vi "daq calib.vi"() -> ()   [LabVIEW 2010]
doc: "I. Description:\nThis example demonstrates how to take a single Measurement (Sample) from an Analog Input Channel.\n\nII. Instructions for Running:\n1. Select the Physical Channel to correspond to where your signal is input on the DAQ device.\n2. Enter the Minimum and Maximum Voltage Ranges\nNote: For better accuracy try to match the Input Ranges to the expected voltage level of the measured signal.\nNote: Use the Gen Voltage Update example to provide a signal on your DAQ device to measure.\n\nIII. Block Diagram Steps:\n1. Create an Analog Input Voltage Channel.\n2. Use the Read VI to Measure 1 Sample from 1 Channel on the Data\nAcquisition Card. Set a timeout so an error is returned if the sample\nis not returned in the specified time limit\n3. Call the Clear Task VI to clear the Task.\n4. Use the popup dialog box to display an error if any.\n\nIV. I/O Connections Overview:\nMake sure your signal input terminal matches the Physical Channel I/O Control."
uses:
  <vilib>/sound2/lvsound2.llb/Sound Data Format.ctl
  <vilib>/Utility/error.llb/DialogType.ctl
  <vilib>/sound2/lvsound2.llb/Sound Output Task ID.ctl
  <vilib>/DAQmx/read.llb/DAQmx Read (Analog DBL 1Chan 1Samp).vi
  <vilib>/DAQmx/write.llb/DAQmx Write (Analog DBL 1Chan 1Samp).vi
  <vilib>/DAQmx/create/channels.llb/DAQmx Create Channel (AI-Voltage-Basic).vi
  <vilib>/DAQmx/create/channels.llb/DAQmx Create Channel (AO-Voltage-Basic).vi
  <vilib>/Utility/file.llb/Write To Spreadsheet File (DBL).vi
  <vilib>/daqmx/miscellaneous.llb/DAQmx Fill In Error Info.vi
  <vilib>/Analysis/NI_AALBase.lvlib
panel:
  out "Vez #":i32
  out "Paso #":i32
  in  "DAC Paso":dbl step=0.001 format="%0.3f"
  in  "DAC Hasta":dbl step=0.001 format="%0.3f"
  in  "DAC Desde":dbl step=0.001 format="%0.3f"
  in  "tiempo entre pasos (ms)":dbl
  in  "Sound Paso":dbl step=0.001 format="%0.3f"
  in  "Sound Hasta":dbl step=0.001 format="%0.3f"
  in  "Sound Desde":dbl step=0.001 format="%0.3f"
  in  "DAC (T) / Sound (F)":bool
  in  "Sound Controls":T2={"device ID"=0, "sound format"={"sample rate (S/s)"=44000.0, "number of channels"=2, "bits per sample"=16}, "time (ms)"=200.0}
  out "Numeric":u32
  in  "Corre":bool
  in  "N":i32
  in  "Maximum Value 2":dbl=10.0 caption="Maximum Value" format="%.2f"
  in  "Minimum Value 2":dbl=-10.0 caption="Minimum Value" format="%0.2f"
  out "In Range?":bool
  in  "Physical Channel 2":tag="Dev1/ai0" caption="Physical Channel"
  in  "stop":bool
  in  "Maximum Value":dbl=10.0 format="%.2f"
  in  "Minimum Value":dbl=-10.0 format="%0.2f"
  in  "Physical Channel":tag="Dev1/ai0"
  # "Channel Parameters"
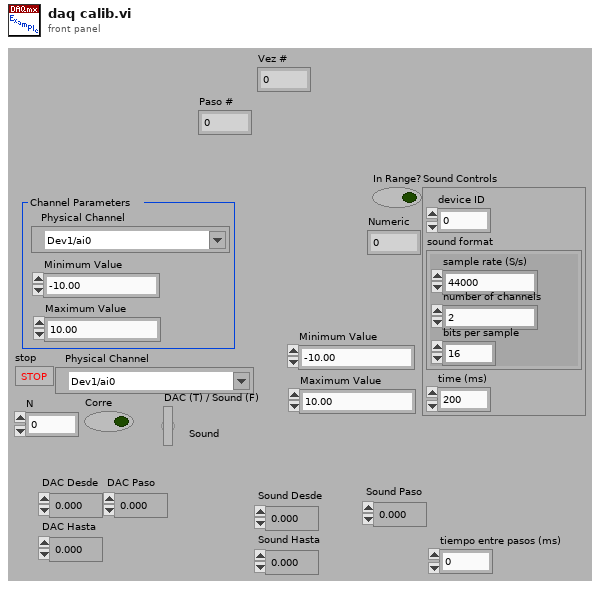
[diagram p1: front panel]
types:
  T1 = typedef "Sound Data Format.ctl" = cluster{"sample rate (S/s)":dbl, "number of channels":i32, "bits per sample":i32}
  T2 = cluster{"device ID":u32, "sound format":T1, "time (ms)":dbl}
  T3 = typedef "Sound Output Task ID.ctl" = u32
  T4 = cluster{"task ID":T3, "error":errorcluster, "sound format":T1}
  T5 = typedef "DialogType.ctl" = u16
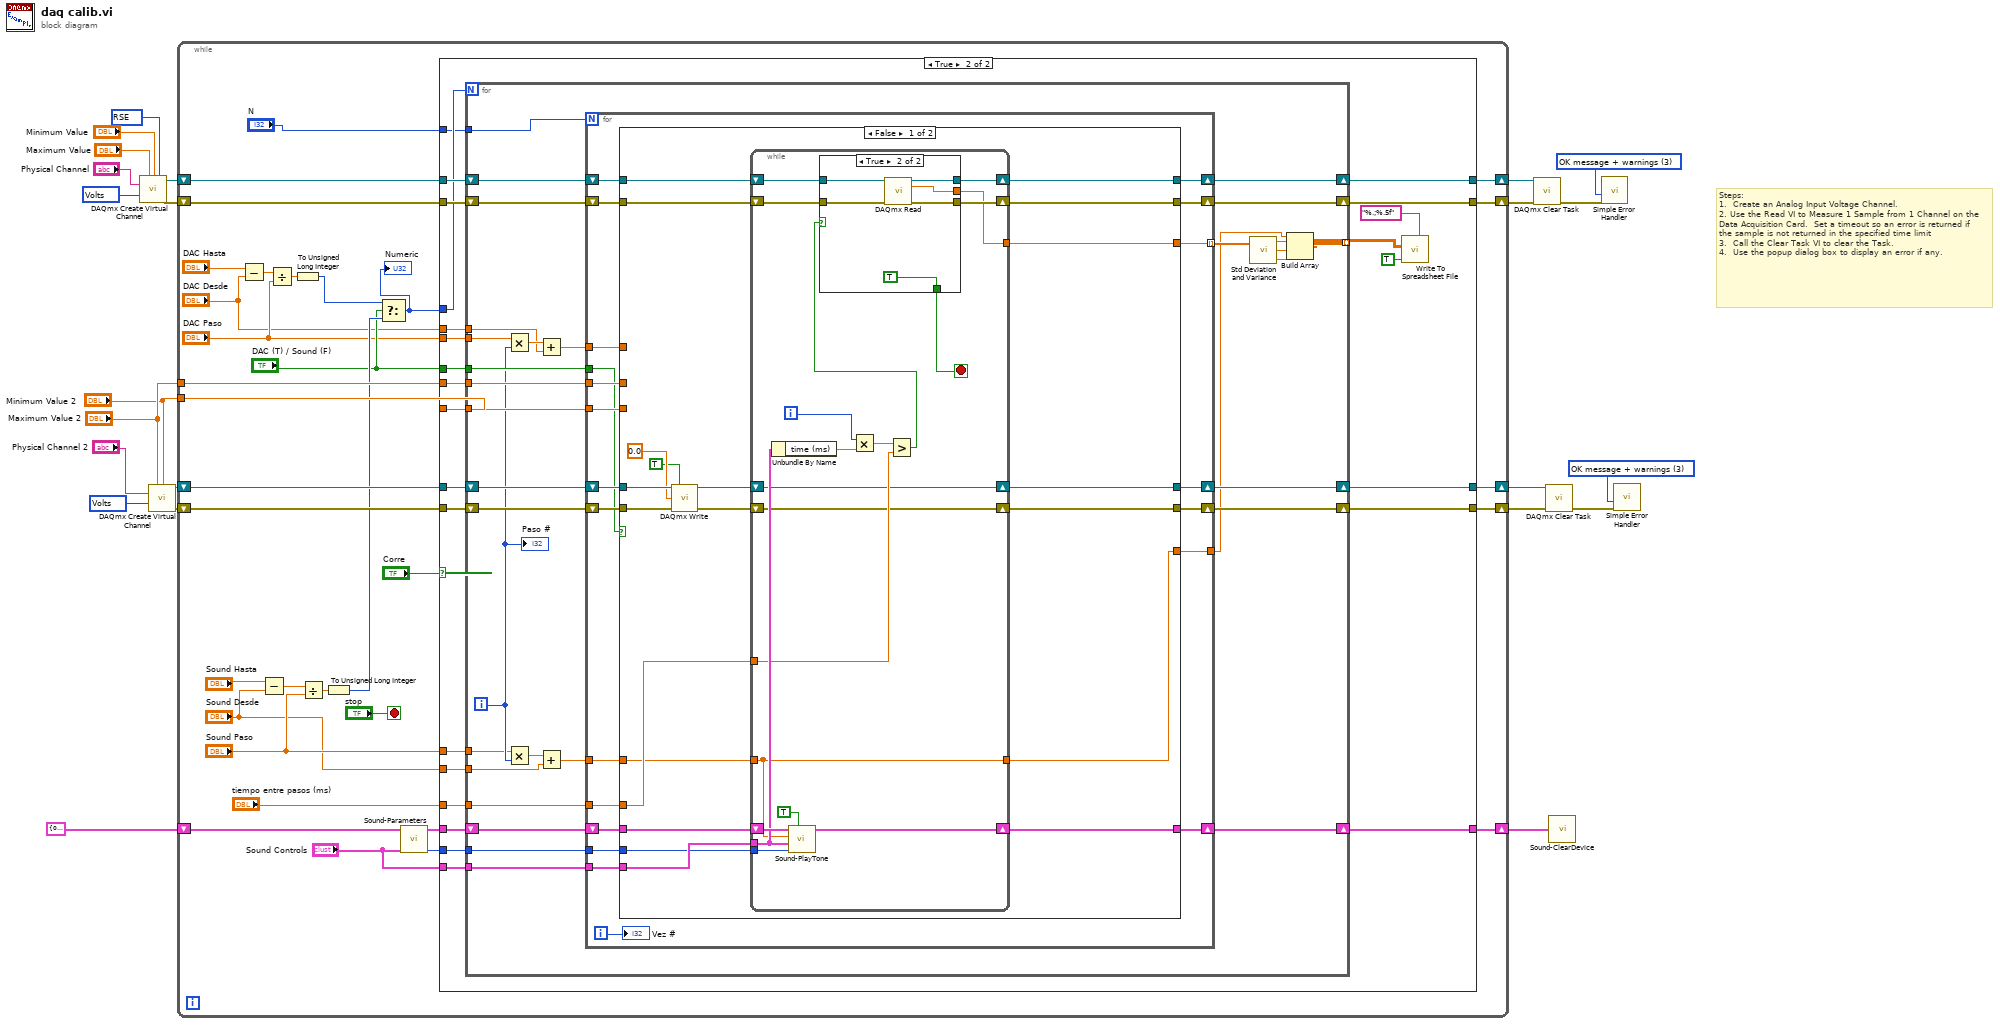
[diagram p0: block diagram]
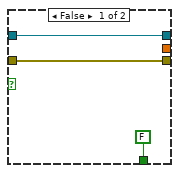
[diagram p3: hidden frame]
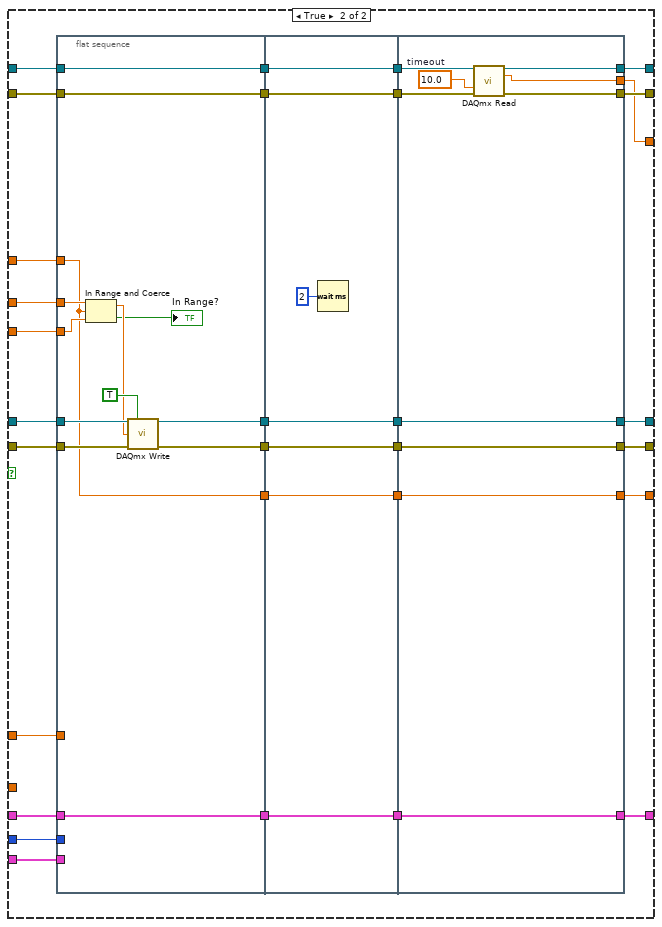
[diagram p4: hidden frame]
diagram:
  w5 = 10083 items=["default"=-1, "RSE"=10083, "NRSE"=10078, "Differential"=10106, "Pseudodifferential"=12529] ("input terminal configuration")
  w8 = 10348 items=["Volts"=10348, "From Custom Scale"=10065] ("units")
  w9 = 10348 items=["Volts"=10348, "From Custom Scale"=10065] ("units")
  w13 = T5 3 items=["no dialog", "OK message", "continue or stop message", "OK message + warnings", "continue/stop + warnings"] ("type of dialog (OK msg:1)")
  w20 = T5 3 items=["no dialog", "OK message", "continue or stop message", "OK message + warnings", "continue/stop + warnings"] ("type of dialog (OK msg:1)")
  # "Steps: \n1.  Create an Analog Input Voltage Channel. \n2. Use the Read VI to Measure 1 Sample from 1 Channel on the Data Acquisition Card.  Set a timeout so an error is returned if the sample is not returned in the specified time limit\n3.  Call the Clear Task VI to clear the Task.\n4.  Use the popup dialog box to display an error if any."
  n1 = call-poly <vilib>:"DAQmx Create Virtual Channel.vi"("maximum value"="Maximum Value", "minimum value"="Minimum Value", "input terminal configuration"=w5, "physical channels"="Physical Channel", "units"=w9) -> ("task out"=w22:refnum<k21>, "error out"=w21:errorcluster)  [unwired: 9 in]
  n2 = call-poly <vilib>:"DAQmx Create Virtual Channel.vi"("maximum value"="Maximum Value 2", "minimum value"="Minimum Value 2", "physical channels"="Physical Channel 2", "units"=w8) -> ("task out"=w15:refnum<k21>, "error out"=w14:errorcluster)  [unwired: 10 in]
  n3 = while {
    shift-right: [w50] -> w19
    shift-left: w22 -> [w53]
    shift-right: [w51] -> w18
    shift-left: w21 -> [w52]
    shift-right: [w49] -> w11
    shift-left: w15 -> [w55]
    shift-right: [w48] -> w10
    shift-left: w14 -> [w54]
    tunnel: "Maximum Value 2" -> [w47]
    tunnel: "Minimum Value 2" -> [w46]
    shift-right: [w42] -> w1
    shift-left: T4 {"task ID"=0, "error"={"status"=TRUE, "code"=0, "source"=""}, "sound format"={"sample rate (S/s)"=0.0, "number of channels"=0, "bits per sample"=0}} ("Sound Device OUT") -> [w44]
    stop <- "stop" stop-if-true
    n4 = Subtract(x="DAC Hasta", y="DAC Desde") -> (x-y=w29:dbl)
    n5 = Subtract(x="Sound Hasta", y="Sound Desde") -> (x-y=w38:dbl)
    n6 = Divide(x=w29, y="DAC Paso") -> (x/y=w28:dbl)
    n7 = To Unsigned Long Integer(number=w28) -> (unsigned 32bit integer=w27:u32)
    n8 = Divide(x=w38, y="Sound Paso") -> (x/y=w37:dbl)
    n9 = To Unsigned Long Integer(number=w37) -> (unsigned 32bit integer=w32:u32)
    n10 = Select(t=w27, s="DAC (T) / Sound (F)", f=w32) -> (s? t:f=w39:u32)
    "Numeric" <- w39
    n11 = call "Sound-Parameters.vi"("Sound Controls"="Sound Controls", "Sound Device IN"=w44) -> ("#samples"=w41:u32, "Sound Device OUT"=w43:T4)  [unwired: 3 in, 1 out]
    n12 = case shown="True" "Corre" {
      tunnel: w55 -> [w59 w86]
      tunnel: w54 -> [w58 w85]
      tunnel: w53 -> [w61 w84]
      tunnel: w52 -> [w60 w83]
      tunnel: [w60 w82] -> w51
      tunnel: [w61 w81] -> w50
      tunnel: [w59 w80] -> w49
      tunnel: [w58 w79] -> w48
      tunnel: w47 -> [_ w78]
      tunnel: w46 -> [_ w77]
      tunnel: w39 -> [_ w76]
      tunnel: "DAC Paso" -> [_ w75]
      tunnel: "DAC Desde" -> [_ w74]
      tunnel: "N" -> [_ w73]
      tunnel: "DAC (T) / Sound (F)" -> [_ w69]
      tunnel: w43 -> [w57 w68]
      tunnel: [w57 w67] -> w42
      tunnel: w41 -> [_ w66]
      tunnel: "Sound Controls" -> [_ w65]
      tunnel: "Sound Paso" -> [_ w64]
      tunnel: "Sound Desde" -> [_ w63]
      tunnel: "tiempo entre pasos (ms)" -> [_ w62]
      frame False {
      }
      frame True {
        n13 = for {
          N: w76 -> [_]
          tunnel: w78 -> [w110]
          tunnel: w77 -> [w109]
          shift-right: [w114] -> w82
          shift-left: w83 -> [w115]
          shift-right: [w113] -> w81
          shift-left: w84 -> [w116]
          shift-right: [w112] -> w80
          shift-left: w86 -> [w118]
          shift-right: [w111] -> w79
          shift-left: w85 -> [w117]
          tunnel: w75 -> [w107]
          tunnel: w74 -> [w106]
          tunnel: w73 -> [w105]
          tunnel: [w103] -> w72 mode=indexing
          tunnel: w69 -> [w97]
          shift-right: [w95] -> w67
          shift-left: w68 -> [w96]
          tunnel: w66 -> [w94]
          tunnel: w65 -> [w93]
          tunnel: w64 -> [w90]
          tunnel: w63 -> [w89]
          tunnel: w62 -> [w87]
          i -> [w91]
          n14 = Multiply(x=w107, y=w91) -> (x*y=w108:dbl)
          n15 = Multiply(x=w90, y=w91) -> (x*y=w92:dbl)
          n16 = Add(x=w108, y=w106) -> (x+y=w99:dbl)
          n17 = Add(x=w92, y=w89) -> (x+y=w88:dbl)
          n18 = for {
            N: w105 -> [_]
            tunnel: w110 -> [w131]
            tunnel: w109 -> [w130]
            shift-right: [w134] -> w113
            shift-left: w116 -> [w137]
            shift-right: [w135] -> w114
            shift-left: w115 -> [w136]
            shift-right: [w133] -> w112
            shift-left: w118 -> [w139]
            shift-right: [w132] -> w111
            shift-left: w117 -> [w138]
            tunnel: w99 -> [w129]
            tunnel: [w128] -> w102 mode=indexing
            tunnel: [w127] -> w98
            tunnel: w97 -> [w120]
            shift-right: [w125] -> w95
            shift-left: w96 -> [w126]
            tunnel: w94 -> [w124]
            tunnel: w93 -> [w123]
            tunnel: w88 -> [w122]
            tunnel: w87 -> [w121]
            i -> [w119]
            n19 = case shown="False" w120 {
              tunnel: w139 -> [w142 w205]
              tunnel: w138 -> [w143 w204]
              tunnel: w137 -> [w157 w203]
              tunnel: w136 -> [w155 w202]
              tunnel: [w154 w201] -> w135
              tunnel: [w156 w200] -> w134
              tunnel: [w147 w199] -> w133
              tunnel: [w148 w198] -> w132
              tunnel: w131 -> [_ w197]
              tunnel: w130 -> [_ w196]
              tunnel: w129 -> [_ w195]
              tunnel: [w149 w194] -> w128
              tunnel: [w146 w193] -> w127
              tunnel: w126 -> [w159 w192]
              tunnel: [w158 w191] -> w125
              tunnel: w124 -> [w152 w190]
              tunnel: w123 -> [w153 w189]
              tunnel: w122 -> [w150 w188]
              tunnel: w121 -> [w151 _]
              frame False {
                n20 = call-poly <vilib>:"DAQmx Write.vi"("task/channels in"=w142, "auto start"=TRUE, "data"=0.0, "error in"=w143) -> ("task out"=w145:refnum<k21>, "error out"=w144:errorcluster)  [unwired: 9 in, 1 out]
                n21 = while {
                  tunnel: w151 -> [w170]
                  tunnel: w150 -> [w160]
                  tunnel: w153 -> [w172]
                  tunnel: w152 -> [w174]
                  shift-right: [w175] -> w156
                  shift-left: w157 -> [w176]
                  shift-right: [w177] -> w158
                  shift-left: w159 -> [w178]
                  shift-right: [w167] -> w154
                  shift-left: w155 -> [w166]
                  tunnel: [w165] -> w149
                  shift-right: [w163] -> w147
                  shift-left: w145 -> [w163]
                  shift-right: [w164] -> w148
                  shift-left: w144 -> [w164]
                  tunnel: [w160] -> w146
                  i -> [w161]
                  stop <- w169 stop-if-true
                  n22 = Unbundle By Name(w172) -> ("time (ms)"=w162:dbl)
                  n23 = call "Sound-PlayTone.vi"("sound?"=TRUE ("DAQ?"), "# samples"=w174, "Sound Controls"=w172, "Frecuencia"=w160, "Sound Device IN"=w178) -> ("Sound Device OUT"=w177:T4)  [unwired: 3 in, 1 out]
                  n24 = Multiply(x=w161, y=w162) -> (x*y=w171:dbl)
                  n25 = Greater?(x=w171, y=w170) -> (0:w168:bool)
                  n26 = case shown="True" w168 {
                    tunnel: w176 -> [w181 w187]
                    tunnel: [w181 w186] -> w175
                    tunnel: [FALSE ("Streeam") TRUE ("Streeam")] -> w169
                    tunnel: [w179 w184] -> w167
                    tunnel: w166 -> [w179 w183]
                    tunnel: [_ w182] -> w165
                    frame False {
                    }
                    frame True {
                      n27 = call-poly <vilib>:"DAQmx Read.vi"("task/channels in"=w187, "error in"=w183) -> ("task out"=w186:refnum<k21>, "data"=w182:dbl, "error out"=w184:errorcluster)  [unwired: 11 in]
                    }
                  }
                }
              }
              frame True {
                n28 = flat-sequence {
                  tunnel: w205 -> [w228]
                  tunnel: w204 -> [w227]
                  tunnel: [w230] -> w217
                  tunnel: w203 -> [w230]
                  tunnel: w202 -> [w229]
                  tunnel: [w229] -> w216
                  tunnel: [w226] -> w215
                  tunnel: [w225] -> w214
                  tunnel: w197 -> [w224]
                  tunnel: w196 -> [w223]
                  tunnel: w195 -> [w222]
                  tunnel: [w222] -> w213
                  tunnel: w192 -> [w221]
                  tunnel: [w221] -> w212
                  tunnel: w190 -> [_]
                  tunnel: w189 -> [_]
                  tunnel: w188 -> [_]
                  tunnel: w217 -> [w237]
                  tunnel: [w237] -> w211
                  tunnel: w216 -> [w236]
                  tunnel: [w236] -> w210
                  tunnel: w215 -> [w235]
                  tunnel: [w235] -> w209
                  tunnel: w214 -> [w234]
                  tunnel: [w234] -> w208
                  tunnel: w213 -> [w233]
                  tunnel: [w233] -> w207
                  tunnel: [w232] -> w206
                  tunnel: w212 -> [w232]
                  tunnel: w211 -> [w246]
                  tunnel: w210 -> [w245]
                  tunnel: [w244] -> w201
                  tunnel: [w243] -> w200
                  tunnel: w209 -> [w242]
                  tunnel: [w242] -> w199
                  tunnel: w208 -> [w241]
                  tunnel: [w241] -> w198
                  tunnel: [w240] -> w194
                  tunnel: w207 -> [w239]
                  tunnel: [w239] -> w193
                  tunnel: [w238] -> w191
                  tunnel: w206 -> [w238]
                  frame #0 {
                    n29 = In Range and Coerce(upper limit=w224, x=w222, lower limit=w223) -> (coerced(x)=w219:dbl, In Range?=→"In Range?":bool)
                    n30 = call-poly <vilib>:"DAQmx Write.vi"("task/channels in"=w228, "auto start"=TRUE, "data"=w219, "error in"=w227) -> ("task out"=w226:refnum<k21>, "error out"=w225:errorcluster)  [unwired: 9 in, 1 out]
                  }
                  frame #1 {
                    n31 = Wait (ms)(milliseconds to wait=u32 2) -> ()  [unwired: 1 out]
                  }
                  frame #2 {
                    w247 = 10.0  # timeout
                    n32 = call-poly <vilib>:"DAQmx Read.vi"("task/channels in"=w246, "timeout"=w247, "error in"=w245) -> ("task out"=w243:refnum<k21>, "data"=w240:dbl, "error out"=w244:errorcluster)  [unwired: 10 in]
                  }
                }
              }
            }
            "Vez #" <- w119
          }
          n33 = call <vilib>:"Std Deviation and Variance.vi"("X"=w102) -> ("mean"=w104:dbl, "standard deviation"=w101:dbl, "variance"=w100:dbl)  [unwired: 1 in]
          n34 = Build Array(w98, w104, w101, w100) -> (w103:dbl[])
          "Paso #" <- w91
        }
        n35 = call-poly <vilib>:"Write To Spreadsheet File.vi"("format (%.3f)"="%.;%.5f", "append to file? (new file:F)"=TRUE, "2D data"=w72) -> ()  [unwired: 5 in, 1 out]
      }
    }
  }
  n36 = call <vilib>:"DAQmx Clear Task.vi"("task in"=w19, "error in"=w18) -> ("error out"=w17:errorcluster)  [unwired: 13 in]
  n37 = call <vilib>:"DAQmx Clear Task.vi"("task in"=w11, "error in"=w10) -> ("error out"=w12:errorcluster)  [unwired: 13 in]
  n38 = call "Sound-ClearDevice.vi"("Sound Device OUT"=w1) -> ()
  n39 = call <vilib>:"Simple Error Handler.vi"("type of dialog (OK msg:1)"=w20, "error in (no error)"=w17) -> ()  [unwired: 3 in, 5 out]
  n40 = call <vilib>:"Simple Error Handler.vi"("type of dialog (OK msg:1)"=w13, "error in (no error)"=w12) -> ()  [unwired: 3 in, 5 out]
